vi "GetBitfile.vi"(8 "error in (no error)":errorcluster, 9 "system info":T1, 11 "bitfile dir":path) -> (0 "error out":errorcluster, 2 "error":string, 3 "bitfile":path, 5 "found":bool)   [LabVIEW 2017, in "EmsaFPGABitfileManager.lvlib"]
uses:
  <vilib>/addons/InsightCM/Devices/Shared/Emsa/EmsaFPGABifileManager/EmsaFPGABitfileManager.lvlib
  <vilib>/addons/cRIODetectHW/control/SystemHW.ctl
  <vilib>/addons/cRIODetectHW/control/cRIO Product Info.ctl
  <vilib>/addons/cRIODetectHW/cRIODetectHW.lvlib
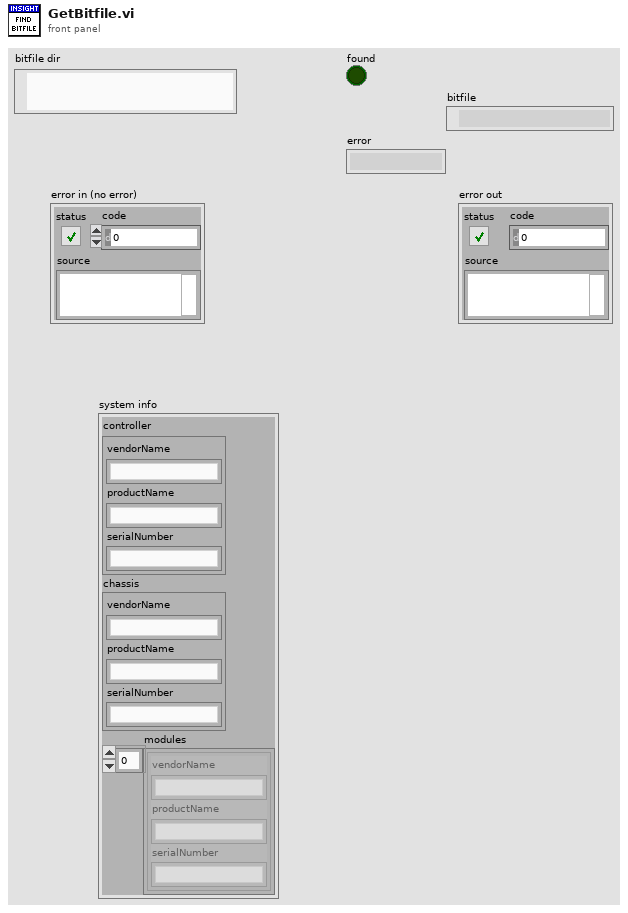
[diagram p1: front panel]
types:
  T1 = typedef "cRIODetectHW.lvlib/SystemHW.ctl" = cluster{"controller":T2, "chassis":T2, "modules":T2[]}
  T2 = typedef "cRIODetectHW.lvlib/cRIO Product Info.ctl" = cluster{"vendorName":string, "productName":string, "serialNumber":string}
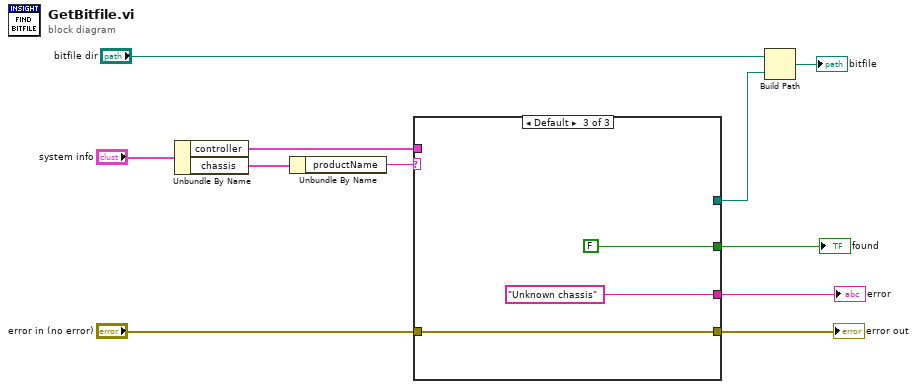
[diagram p0: block diagram]
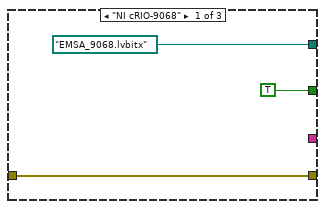
[diagram p2: hidden frame]
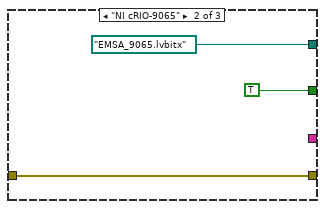
[diagram p3: hidden frame]
diagram:
  n1 = Unbundle By Name("system info") -> ("controller"=w8:T2, "chassis"=w10:T2)
  n2 = Unbundle By Name(w10) -> ("productName"=w9:string)
  n3 = case shown="Default" w9 {
    tunnel: w8 -> [_ _ _]
    tunnel: [path "EMSA_9068.lvbitx" path "EMSA_9065.lvbitx" _] -> w4
    tunnel: [w13 w17 w20] -> w7
    tunnel: "error in (no error)" -> [w13 w17 w20]
    tunnel: [_ _ "Unknown chassis" ("source")] -> w2
    tunnel: [TRUE TRUE FALSE] -> w1
    frame "NI cRIO-9068" {
    }
    frame "NI cRIO-9065" {
    }
    frame Default {
    }
  }
  "error out" <- w7
  "error" <- w2
  "found" <- w1
  n4 = Build Path(base path="bitfile dir", name or relative path=w4) -> (appended path=→"bitfile":path)
